vi "LabvolutionSubmoduleCheck_DisplaySubmoduleInfo.vi"(11 "Project Path in":path) -> ()   [LabVIEW 2018]
panel:
  in  "Submodule Status":bool
  in  "Reset Submodules":bool
  in  "Pull Updates":bool
  in  "Fetch Updates":bool
  out "Project Path":path
  out "Submodules within project":string
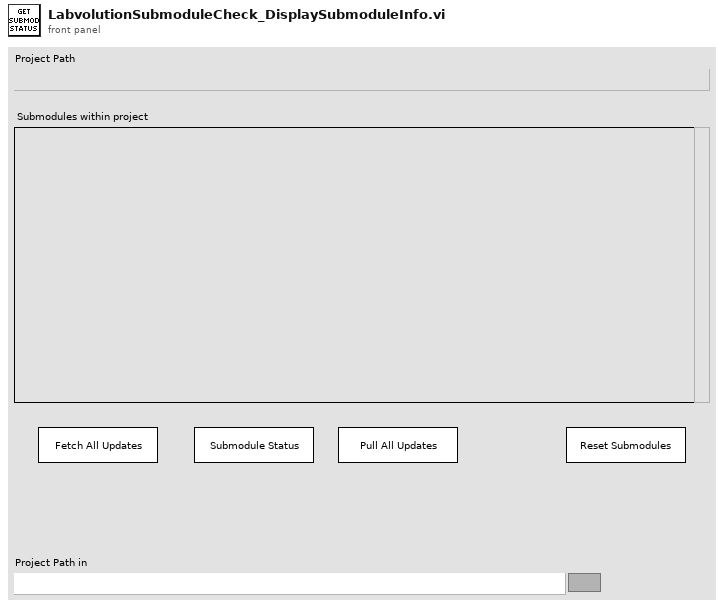
[diagram p1: front panel]
types:
  T1 = enum32{"Invalid", "Standard", "Closed", "Hidden", "Minimized", "Maximized"}
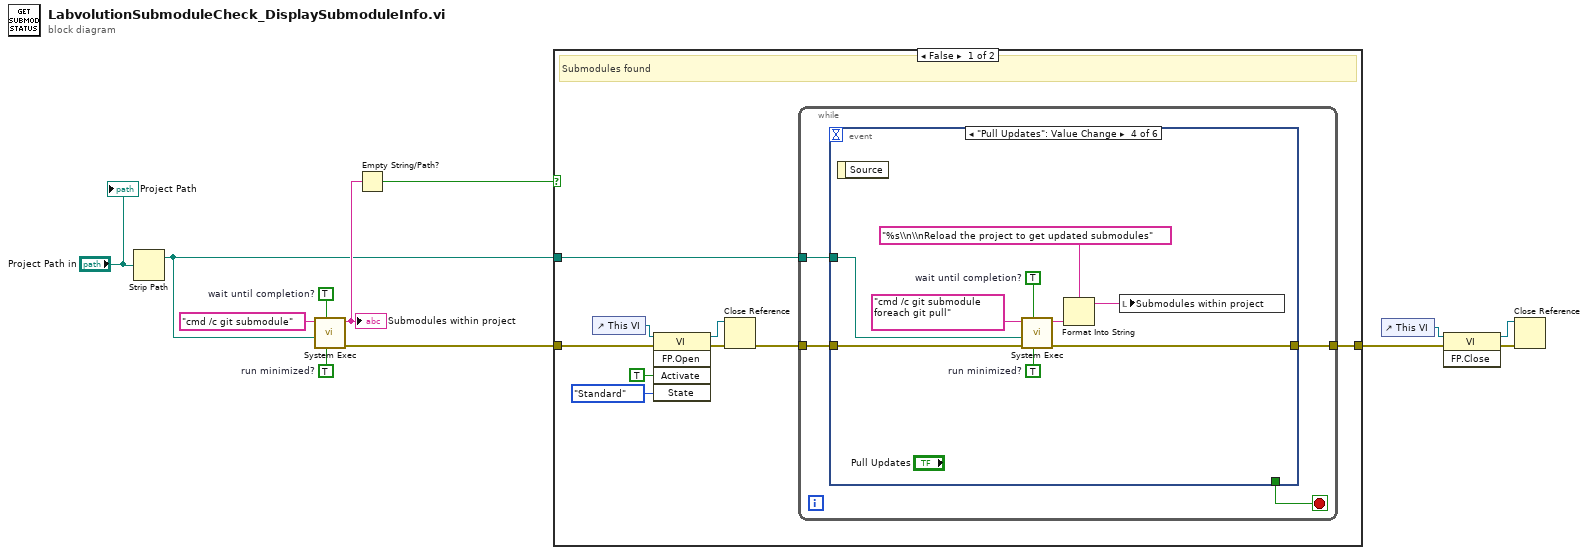
[diagram p0: block diagram]
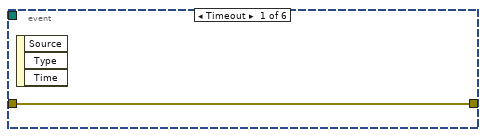
[diagram p2: hidden frame]
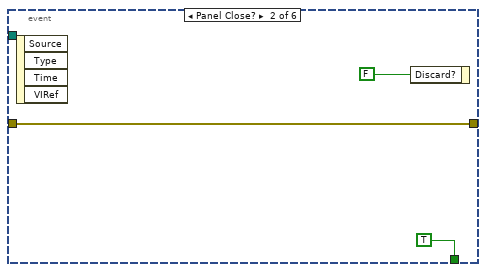
[diagram p3: hidden frame]
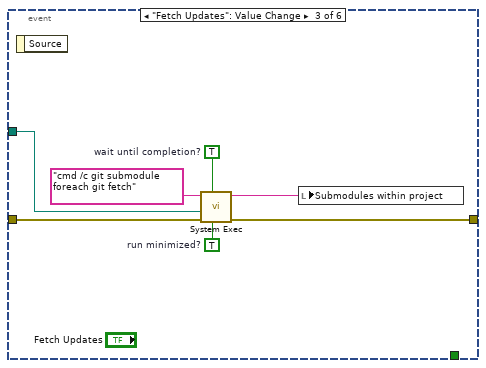
[diagram p4: hidden frame]
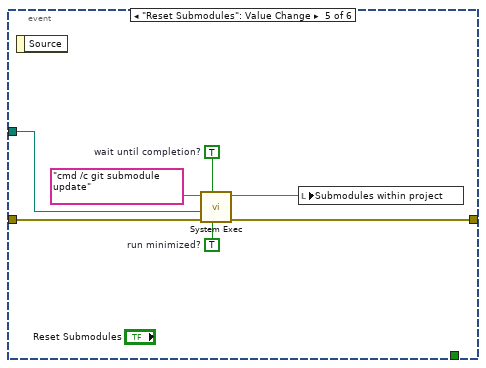
[diagram p5: hidden frame]
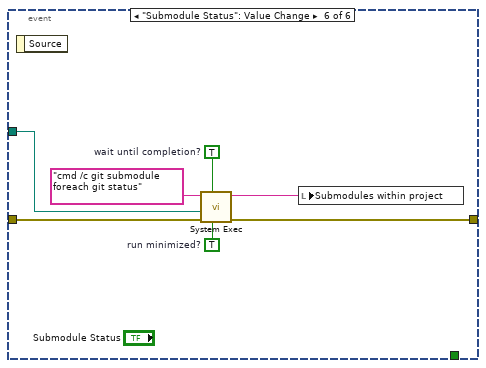
[diagram p6: hidden frame]
diagram:
  w9 = TRUE  # run minimized?
  w10 = TRUE  # wait until completion?
  n1 = Strip Path(path="Project Path in") -> (stripped path=w3:path)  [unwired: 1 out]
  n2 = call <vilib>:"System Exec.vi"("run minimized? (F)"=w9, "wait until completion? (T)"=w10, "working directory"=w3, "command line"="cmd /c git submodule") -> ("error out"=w8:errorcluster, "standard output"=w5:string)  [unwired: 4 in, 2 out]
  "Submodules within project" <- w5
  n3 = Empty String/Path?(string/path=w5) -> (empty?=w4:bool)
  n4 = case shown="False" w4 {
    tunnel: w8 -> [w21 w60]
    tunnel: [w17 w60] -> w6
    tunnel: w3 -> [w16 _]
    frame False {
      # "Submodules found"
      n5 = control-ref of="This VI"() -> (w20:refnum<vi>)
      n6 = invoke class="VI" method="FP.Open"(reference=w20, error in=w21, "Activate"=TRUE ("Activate?"), "State"=T1."Standard") -> (reference out=w13:refnum<vi>, error out=w15:errorcluster)  [unwired: 1 in, 3 out]
      n7 = Close Reference(reference=w13, error in (no error)=w15) -> (error out=w14:errorcluster)
      n8 = while {
        tunnel: w14 -> [w24]
        tunnel: [w23] -> w17
        tunnel: w16 -> [w22]
        stop <- w25 stop-if-true
        n9 = event shown="[3] \"Pull Updates\": Value Change" {
          selector: _ -> [_ _ _ _ _ _]
          dyn-events: _ -> [_ _ _ _ _ _]
          timeout: _ -> [_ _ _ _ _ _]
          tunnel: [_ TRUE _ _ _ _] -> w25
          tunnel: w24 -> [w26 w28 w33 w42 w49 w56]
          tunnel: [w26 w28 w32 w41 w48 w55] -> w23
          tunnel: w22 -> [_ _ w31 w40 w47 w54]
          event Timeout {
            n10 = event-data() -> ()  [unwired: 1 in, 3 out]
          }
          event Panel Close? {
            n11 = event-data() -> ()  [unwired: 1 in, 4 out]
            n12 = event-data("Discard?"=FALSE) -> ()  [unwired: 1 in, 1 out]
          }
          event "Fetch Updates": Value Change {
            w36 = TRUE  # run minimized?
            w35 = TRUE  # wait until completion?
            n13 = event-data() -> ()  [unwired: 1 in, 1 out]
            n14 = call <vilib>:"System Exec.vi"("run minimized? (F)"=w36, "wait until completion? (T)"=w35, "error in (no error)"=w33, "working directory"=w31, "command line"="cmd /c git submodule foreach git fetch") -> ("error out"=w32:errorcluster, "standard output"=w30:string)  [unwired: 3 in, 2 out]
            n15 = local write "Submodules within project"(w30) -> ()
          }
          event "Pull Updates": Value Change {
            w45 = TRUE  # run minimized?
            w44 = TRUE  # wait until completion?
            n16 = event-data() -> ()  [unwired: 1 in, 1 out]
            n17 = call <vilib>:"System Exec.vi"("run minimized? (F)"=w45, "wait until completion? (T)"=w44, "error in (no error)"=w42, "working directory"=w40, "command line"="cmd /c git submodule foreach git pull") -> ("error out"=w41:errorcluster, "standard output"=w38:string)  [unwired: 3 in, 2 out]
            n18 = Format Into String(format string="%s\\n\\nReload the project to get updated submodules", w38) -> (resulting string=w37:string)  [unwired: 2 in, 1 out]
            n19 = local write "Submodules within project"(w37) -> ()
          }
          event "Reset Submodules": Value Change {
            w52 = TRUE  # run minimized?
            w51 = TRUE  # wait until completion?
            n20 = event-data() -> ()  [unwired: 1 in, 1 out]
            n21 = call <vilib>:"System Exec.vi"("run minimized? (F)"=w52, "wait until completion? (T)"=w51, "error in (no error)"=w49, "working directory"=w47, "command line"="cmd /c git submodule update") -> ("error out"=w48:errorcluster, "standard output"=w46:string)  [unwired: 3 in, 2 out]
            n22 = local write "Submodules within project"(w46) -> ()
          }
          event "Submodule Status": Value Change {
            w59 = TRUE  # run minimized?
            w58 = TRUE  # wait until completion?
            n23 = event-data() -> ()  [unwired: 1 in, 1 out]
            n24 = call <vilib>:"System Exec.vi"("run minimized? (F)"=w59, "wait until completion? (T)"=w58, "error in (no error)"=w56, "working directory"=w54, "command line"="cmd /c git submodule foreach git status") -> ("error out"=w55:errorcluster, "standard output"=w53:string)  [unwired: 3 in, 2 out]
            n25 = local write "Submodules within project"(w53) -> ()
          }
        }
      }
    }
    frame True {
      # "Empty submodule string so don't bother running as there are no submodules within the project"
    }
  }
  n26 = control-ref of="This VI"() -> (w7:refnum<vi>)
  n27 = invoke class="VI" method="FP.Close"(reference=w7, error in=w6) -> (reference out=w1:refnum<vi>, error out=w2:errorcluster)  [unwired: 1 in, 1 out]
  n28 = Close Reference(reference=w1, error in (no error)=w2) -> ()  [unwired: 1 out]
  "Project Path" <- "Project Path in"
